vi "Ramp_Conversion.vi"(4 "Offset (0) / nm":dbl, 5 "Sampling rate (20k) / Hz":dbl=20000.0, 6 "Piezo In (0) / V":dbl, 7 "Piezo Sensitivity (1.95) / nm V-1":dbl=1.95, 8 "Error in":errorcluster, 10 "Bias Ramp In (0) / V":dbl[](array[numeric]), 11 "Piezo Ramp In (0) / V":dbl[](array[numeric])) -> (0 "Error Out":errorcluster, 2 "appended array":waveform(dbl)[](array[waveform]))   [LabVIEW 2023]
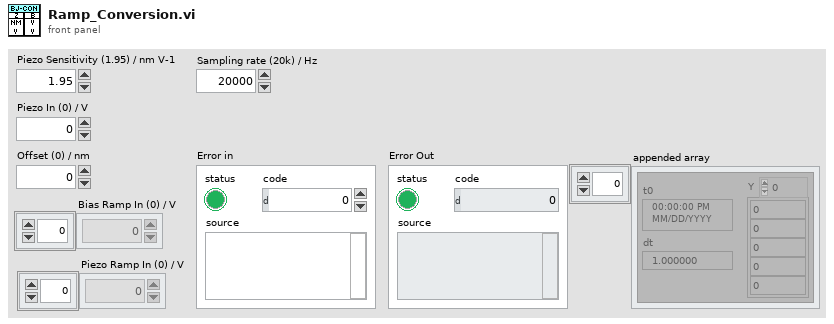
[diagram p1: front panel]
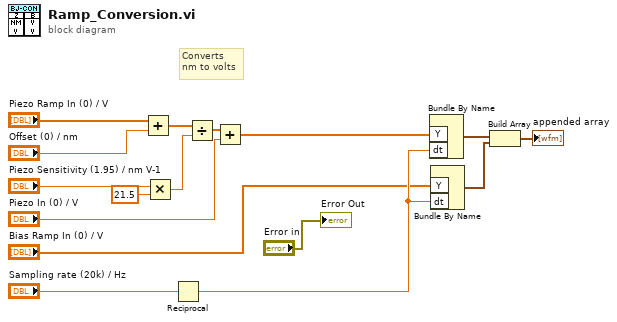
[diagram p0: block diagram]
diagram:
  # "Converts\nnm to volts"
  n1 = Add(x="Piezo Ramp In (0) / V", y="Offset (0) / nm") -> (x+y=w16:dbl[])
  n2 = Multiply(x="Piezo Sensitivity (1.95) / nm V-1", y=21.5) -> (x*y=w9:dbl)
  n3 = Reciprocal(x="Sampling rate (20k) / Hz") -> (1/x=w6:dbl)
  n4 = Divide(x=w16, y=w9) -> (x/y=w15:dbl[])
  n5 = Add(x=w15, y="Piezo In (0) / V") -> (x+y=w5:dbl[])
  n6 = Bundle By Name("Y"=w5, "dt"=w6) -> (w3:waveform(dbl))  [unwired: 1 in]
  n7 = Bundle By Name("Y"="Bias Ramp In (0) / V", "dt"=w6) -> (w2:waveform(dbl))  [unwired: 1 in]
  n8 = Build Array(w3, w2) -> (→"appended array":waveform(dbl)[])
  "Error Out" <- "Error in"
